vi "buildSetTemperature.vi"(8 "error in (no error)":errorcluster, 10 "temperature[°C]":i32, 11 "ICommandBuilder in":refnum<class "ICommandBuilder.lvclass">) -> (0 "error out":errorcluster, 3 "ICommandBuilder out":refnum<class "ICommandBuilder.lvclass">)   [LabVIEW 2023, in "AbstractFactory.lvlib" / "ICommandBuilder.lvclass"]
uses:
  ICommandBuilder.lvclass
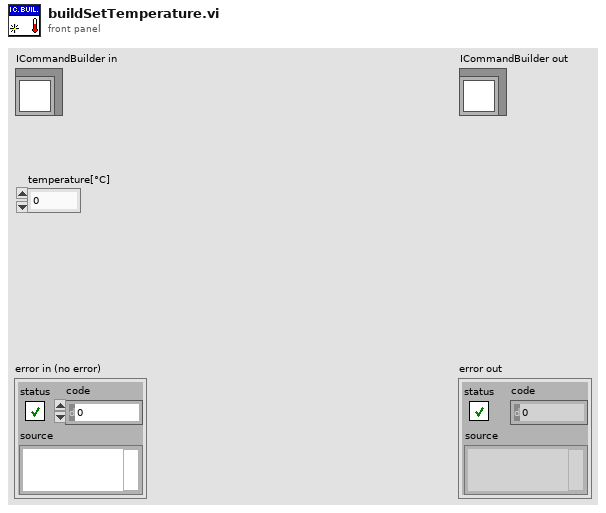
[diagram p1: front panel]
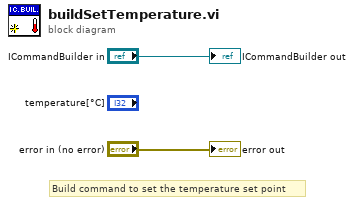
[diagram p0: block diagram]
diagram:
  # "Build command to set the temperature set point"
  "error out" <- "error in (no error)"
  "ICommandBuilder out" <- "ICommandBuilder in"
